vi "VI Server_Open VI Controls Refs_Labels_VI Name Input.vi"(8 "error in (no error)":errorcluster, 11 "VI Name":string) -> (0 "error out":errorcluster, 3 "VI Server Cluster.OUT":T1)   [LabVIEW 2020, in "VI Server Toolkit LV2013.lvlib"]
doc: "Generates the VI Server cluster for VI specified by name. That VI should be loaded into memory."
uses:
  VI Server Toolkit LV2013.lvlib
  VI Server_TypeDefs/VI Server_RefsCluster.ctl
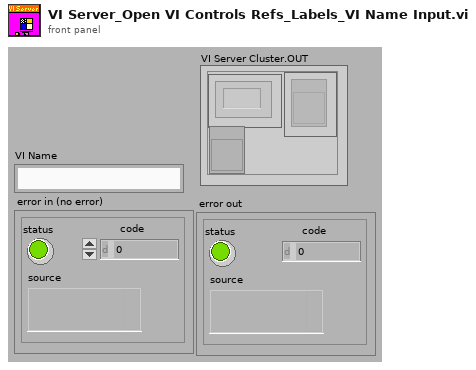
[diagram p1: front panel]
types:
  T1 = typedef "VI Server_RefsCluster.ctl" = cluster{"Labels":string[], "Refs":refnum<vi>[], "VI Ref":refnum<vi>}
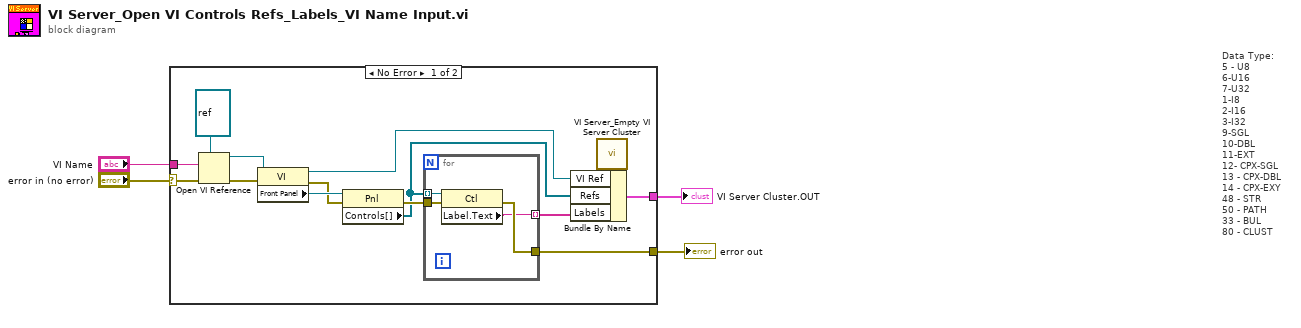
[diagram p0: block diagram]
diagram:
  # "Data Type:\n5 - U8\n6-U16\n7-U32\n1-I8\n2-I16\n3-I32\n9-SGL\n10-DBL\n11-EXT\n12- CPX-SGL\n13 - CPX-DBL\n14 - CPX-EXY\n48 - STR\n50 - PATH\n33 - BUL\n80 - CLUST"
  n1 = case shown="No Error" "error in (no error)" {
    selector: "error in (no error)" -> [w6 w23]
    tunnel: [w14 w23] -> w4
    tunnel: [w11 _] -> w3
    tunnel: "VI Name" -> [w7 _]
    frame No Error {
      n2 = Open VI Reference(type specifier VI Refnum (for type only)=refnum<vi> refnum ("type specifier"), vi path=w7, error in (no error)=w6) -> (vi reference=w12:refnum<vi>, error out=w15:errorcluster)  [unwired: 3 out]
      n3 = property class="VI"(reference=w12, error in=w15) -> (reference out=w9:refnum<vi>, error out=w17:errorcluster, "Front Panel"=w18:refnum<vi>)
      n4 = property class="Pnl"(reference=w18, error in=w17) -> (error out=w16:errorcluster, "Controls[]"=w8:refnum<vi>[])  [unwired: 1 out]
      n5 = for {
        tunnel: w8 -> [w22] mode=indexing
        tunnel: w16 -> [w21]
        tunnel: [w20] -> w14
        tunnel: [w19] -> w10 mode=indexing
        n6 = property class="Ctl"(reference=w22, error in=w21) -> (error out=w20:errorcluster, "Label.Text"=w19:string)  [unwired: 1 out]
      }
      n7 = call "VI Server_Empty VI Server Cluster.vi"() -> ("VI Server Cluster"=w5:T1)  [unwired: 7 in]
      n8 = Bundle By Name(cluster=w5, "VI Ref"=w9, "Refs"=w8, "Labels"=w10) -> (w11:T1)
    }
    frame Error {
    }
  }
  "error out" <- w4
  "VI Server Cluster.OUT" <- w3
